vi "motor_control.vi"(8 "set velocity":dbl format="%.2f", 9 "set position":dbl format="%.2f", 10 "Axis in in":i32, 11 "VISA Refnum in":refnum<visa-resource-name>) -> (0 "actual velocity":dbl format="%.2f", 1 "actual position":dbl format="%.2f", 2 "Axis out":i32=1, 3 "VISA Handle out":refnum<visa-resource-name>)   [LabVIEW 2025]
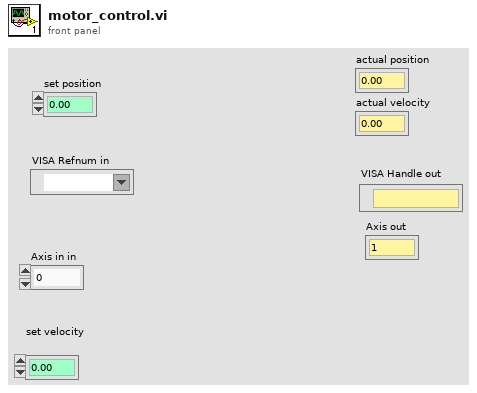
[diagram p1: front panel]
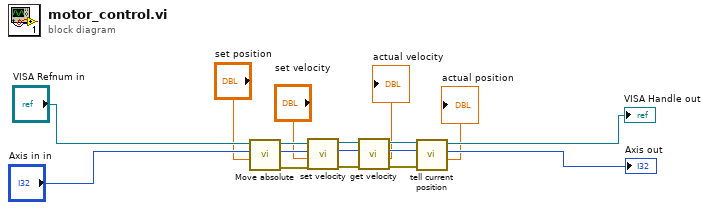
[diagram p0: block diagram]
diagram:
  n1 = call <userlib>:"Move absolute.vi"("New target position (units)"="set position", "Axis in"="Axis in in", "VISA Handle in"="VISA Refnum in") -> ("error out"=w9:errorcluster, "Axis out"=w10:i32, "VISA Handle out"=w11:refnum<visa-resource-name>)  [unwired: 3 in, 1 out]
  n2 = call <userlib>:"set velocity.vi"("error in"=w9, "Velocity value (units/s)"="set velocity", "Axis in"=w10, "VISA Handle in"=w11) -> ("error out"=w5:errorcluster, "Axis out"=w6:i32, "VISA Handle out"=w7:refnum<visa-resource-name>)  [unwired: 2 in, 1 out]
  n3 = call <userlib>:"get velocity.vi"("error in"=w5, "Axis in"=w6, "VISA Handle in"=w7) -> ("error out"=w1:errorcluster, "Velocity value (units/s)"=→"actual velocity":dbl, "Axis out"=w3:i32, "VISA Handle out"=w4:refnum<visa-resource-name>)  [unwired: 2 in, 1 out]
  n4 = call <userlib>:"tell current position.vi"("error in"=w1, "Axis in"=w3, "VISA Handle in"=w4) -> ("Current position (units)"=→"actual position":dbl, "Axis out"=→"Axis out":i32, "VISA Handle out"=→"VISA Handle out":refnum<visa-resource-name>)  [unwired: 2 in, 2 out]
